vi "Stream Basic.vi"() -> ()   [LabVIEW 2009]
panel:
  in  "STREAM_RESOLUTION_INDEX":i32
  in  "STREAM_SETTLING_US":i32
  in  "AIN_ALL_RANGE":dbl=10.0 format="%.3f"
  out "ScansPerRead":i32=500
  out "ConnectionType Out":i32
  out "DeviceType Out":i32
  in  "Identifier":string="10.251.225.90"
  in  "ConnectionType":string="WIFI"
  in  "DeviceType":string="LJM_dtANY"
  in  "NumNames to Scan":i32=4
  out "DeviceScanBacklog":i32
  out "LJMScanBacklog":i32
  out "Data":dbl[][](array[numeric]) format="%.3f"
  out "Waveform Graph":dbl[][](graph)
  in  "Scan List":string[](array[string])=["AIN0", "AIN1", "AIN2", "AIN3"]
  out "# of iterations":i32
  in  "Scan Rate (Hz)":dbl=25.0 format="%.3f"
  in  "stop":bool
  out "Error Message":string="LabJack Error #1263:  LJME_NO_RESPONSE_BYTES_RECEIVED occured at LJM_OpenS.vi"
  # "To remove an element, right-click\non it, select Data Operations =>\nRemove Element.\n\nTo empty an array, right-click\nnear the edge, select Data\nOperations => Empty Array.\n\nOther useful operations:  From the\nOperate menu are \"Make Current\nValues Default\" and \"Reinitialize\nTo Default\"."
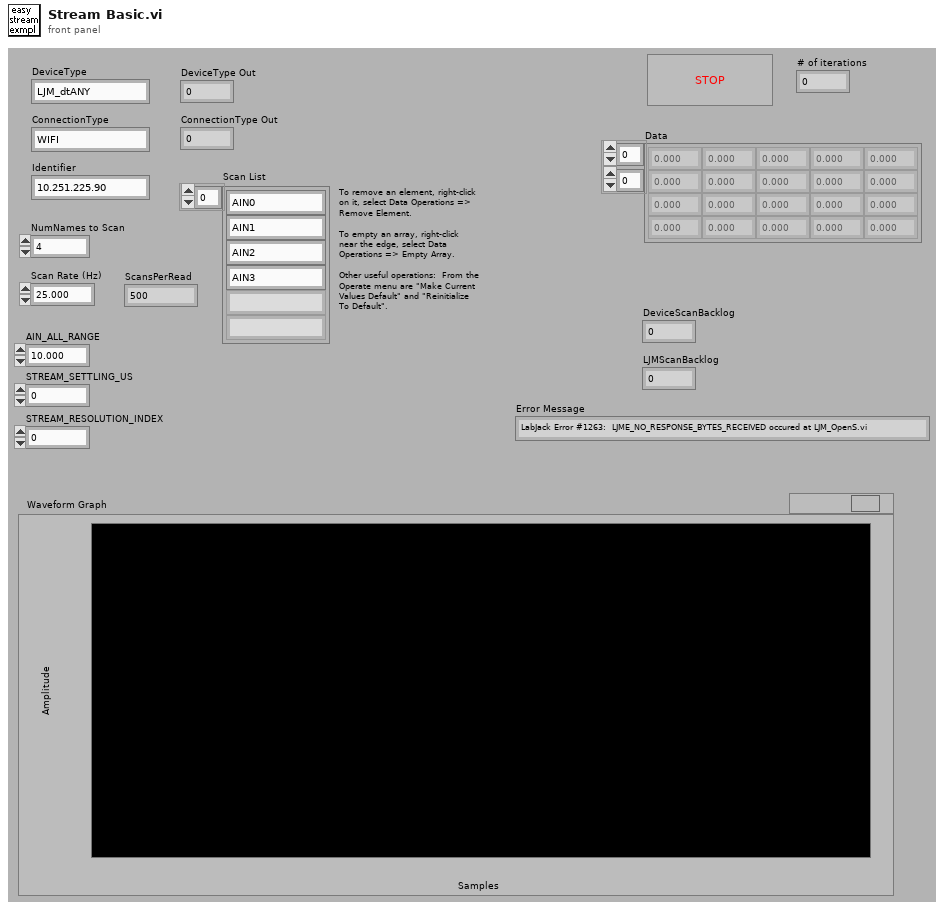
[diagram p1: front panel]
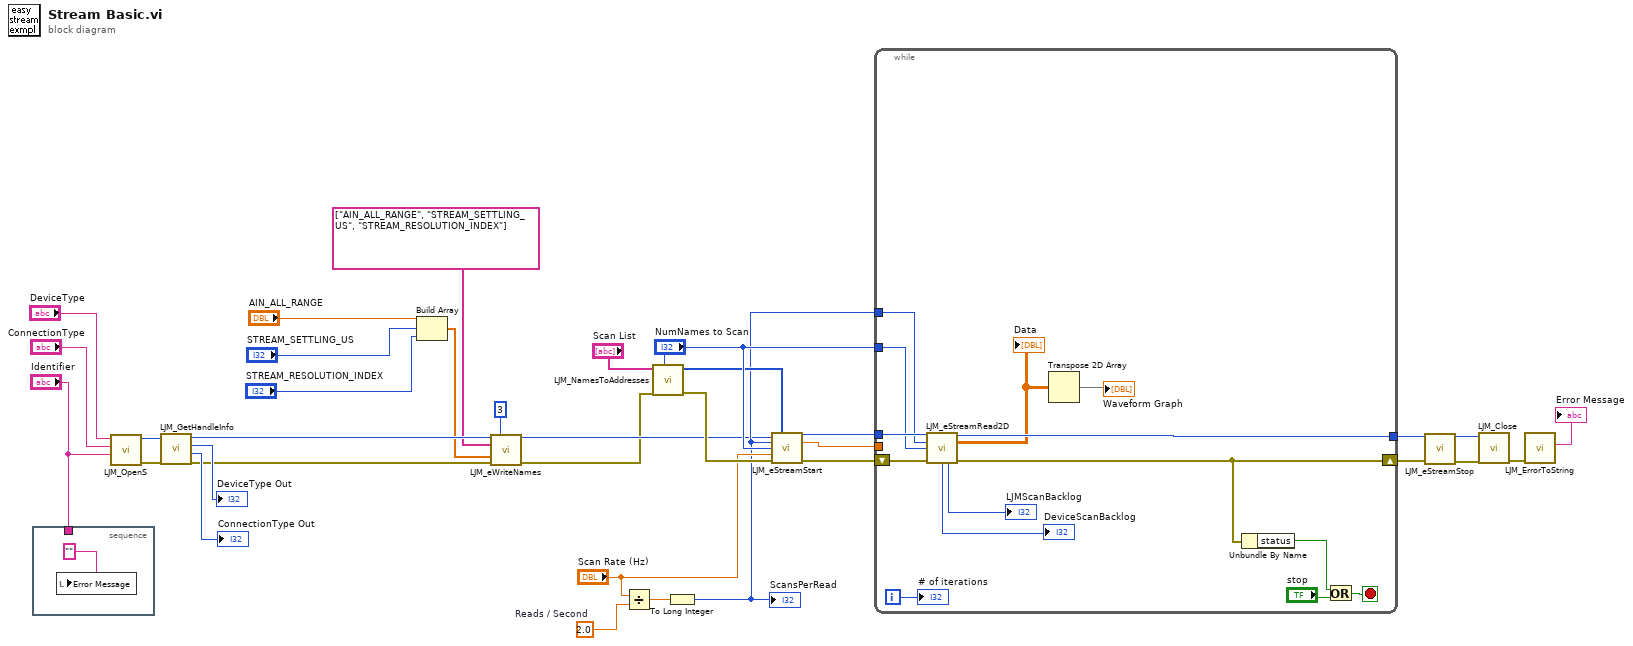
[diagram p0: block diagram]
diagram:
  w13 = 2.0  # Reads / Second
  n1 = stacked-sequence {
    tunnel: "Identifier" -> [_]
    frame #0 {
      n2 = local write "Error Message"("" ("Error Message")) -> ()
    }
  }
  n3 = call <vilib>:"LJM_OpenS.vi"("Identifier"="Identifier", "ConnectionType"="ConnectionType", "DeviceType"="DeviceType") -> ("error out"=w25:errorcluster, "Handle"=w22:i32)  [unwired: 7 in]
  n4 = call <vilib>:"LJM_GetHandleInfo.vi"("error in"=w25, "Handle In"=w22) -> ("error out"=w10:errorcluster, "ConnectionType"=→"ConnectionType Out":i32, "DeviceType"=→"DeviceType Out":i32, "Handle Out"=w9:i32)  [unwired: 2 in, 4 out]
  n5 = Build Array("AIN_ALL_RANGE", "STREAM_SETTLING_US", "STREAM_RESOLUTION_INDEX") -> (w3:dbl[])
  n6 = call <vilib>:"LJM_eWriteNames.vi"("Handle In"=w9, "NumFrames"=3, "aNames"=string[] ["AIN_ALL_RANGE", "STREAM_SETTLING_US", "STREAM_RESOLUTION_INDEX"], "aValuesIn"=w3, "error in"=w10) -> ("Handle Out"=w8:i32, "error out"=w7:errorcluster)  [unwired: 8 in, 1 out]
  n7 = Divide(x="Scan Rate (Hz)", y=w13) -> (x/y=w12:dbl)
  n8 = call <vilib>:"LJM_NamesToAddresses.vi"("NumFrames"="NumNames to Scan", "error in"=w7, "aNames"="Scan List") -> ("error out"=w15:errorcluster, "aAddresses"=w16:i32[])  [unwired: 6 in, 1 out]
  n9 = To Long Integer(number=w12) -> (32bit integer=w11:i32)
  "ScansPerRead" <- w11
  n10 = call <vilib>:"LJM_eStreamStart.vi"("Handle In"=w8, "aScanList"=w16, "ScansPerRead"=w11, "NumAddresses"="NumNames to Scan", "ScanRate"="Scan Rate (Hz)", "error in"=w15) -> ("Handle Out"=w32:i32, "Actual ScanRate"=w33:dbl, "error out"=w34:errorcluster)  [unwired: 7 in]
  n11 = while {
    tunnel: [w42] -> w30
    tunnel: w32 -> [w43]
    tunnel: w33 -> [_]
    shift-left: w34 -> [w44]
    shift-right: [w36] -> w31
    tunnel: w11 -> [w38]
    tunnel: "NumNames to Scan" -> [w37]
    i -> [w46]
    stop <- w47 stop-if-true
    n12 = call <vilib>:"LJM_eStreamRead2D.vi"("Handle In"=w43, "ScansPerRead"=w38, "NumAddresses"=w37, "error in"=w44) -> ("Handle Out"=w42:i32, "aData Out"=w41:dbl[][], "DeviceScanBacklog"=→"DeviceScanBacklog":i32, "LJMScanBacklog"=→"LJMScanBacklog":i32, "error out"=w36:errorcluster)  [unwired: 7 in]
    "Data" <- w41
    n13 = Transpose 2D Array(2D array=w41) -> (transposed array=→"Waveform Graph":dbl[][])
    n14 = Unbundle By Name(w36) -> ("status"=w48:bool)
    n15 = Or(x=w48, y="stop") -> (x .or. y?=w47:bool)
    "# of iterations" <- w46
  }
  n16 = call <vilib>:"LJM_eStreamStop.vi"("Handle In"=w30, "error in"=w31) -> ("Handle Out"=w28:i32, "error out"=w29:errorcluster)  [unwired: 12 in]
  n17 = call <vilib>:"LJM_Close.vi"("error in"=w29, "Handle"=w28) -> ("error out"=w27:errorcluster)  [unwired: 9 in]
  n18 = call <vilib>:"LJM_ErrorToString.vi"("error in"=w27) -> ("String"=→"Error Message":string)  [unwired: 10 in]
